vi "Pixel time analisis viewer.vi"() -> ()   [LabVIEW 2015, in "VIPM2.lvlib"]
uses:
  VIPM2.lvlib
  <vilib>/Analysis/NI_AALBase.lvlib
panel:
  out "Integrated Last event (s)":dbl format="%#.4f s"
  out "Chip Last event (s)":dbl format="%#.4f s"
  out "Chip First event (s)":dbl format="%#.4f s"
  out "Global Last event (s)":dbl format="%#.4f s"
  out "Pixel":u8
  out "Integrated events":i32
  out "Global last event (hex)":u64 format="%.0x"
  out "Global 1st event (hex)":u64 format="%.0x"
  in  "Integration pointer slide":u64(slide) scale=143772870070.0..145064784669.0 scale format="%x"
  out "Total time bar":cluster{u64, u64}(slide) scale=141174816241.0..145064861029.0 scale format="%x"
  in  "Pixel":u8 max=99
  in  "Chip ID":u16 format="%04x"
  out "Barra Load events":i32(slide) scale=-1.0..40000.0
  in  "X scale max.":dbl=150.0 min=0.0 max=1e+29 step=10.0
  in  "X scale min.":dbl=80.0 min=0.0 max=1e+29 step=10.0
  in  "Y scale":dbl=100.0 min=5.0 max=1e+29 step=10.0
  in  "Take image button":bool
  in  "Close button":bool
  out "Total number of events":i32 caption="Total number of events\nCentrals"
  out "data time":string
  in  "ACQ full DATA file path":path caption="File path"
  out "Chip ID":string
  out "Trigger histogram 08":T1(graph)
  out "Trigger histogram 07":T1(graph)
  out "Trigger histogram 06":T1(graph)
  out "Trigger histogram 01":T1(graph)
  out "Trigger histogram 02":T1(graph)
  out "Trigger histogram 03":T1(graph)
  out "Trigger histogram 04":T1(graph)
  out "Trigger histogram 00":T1(graph)
  out "Trigger histogram 05":T1(graph)
  # "Global acquisition time"
  # "03"
  # "04"
  # "05"
  # "Global First acquired event"
  # "Global Last acquired event"
  # "This Chip First event"
  # "This Chip Last event"
  # "02"
  # "00"
  # "01"
  # "Integration slide"
  # "Last integrated event"
  # "08"
  # "07"
  # "06"
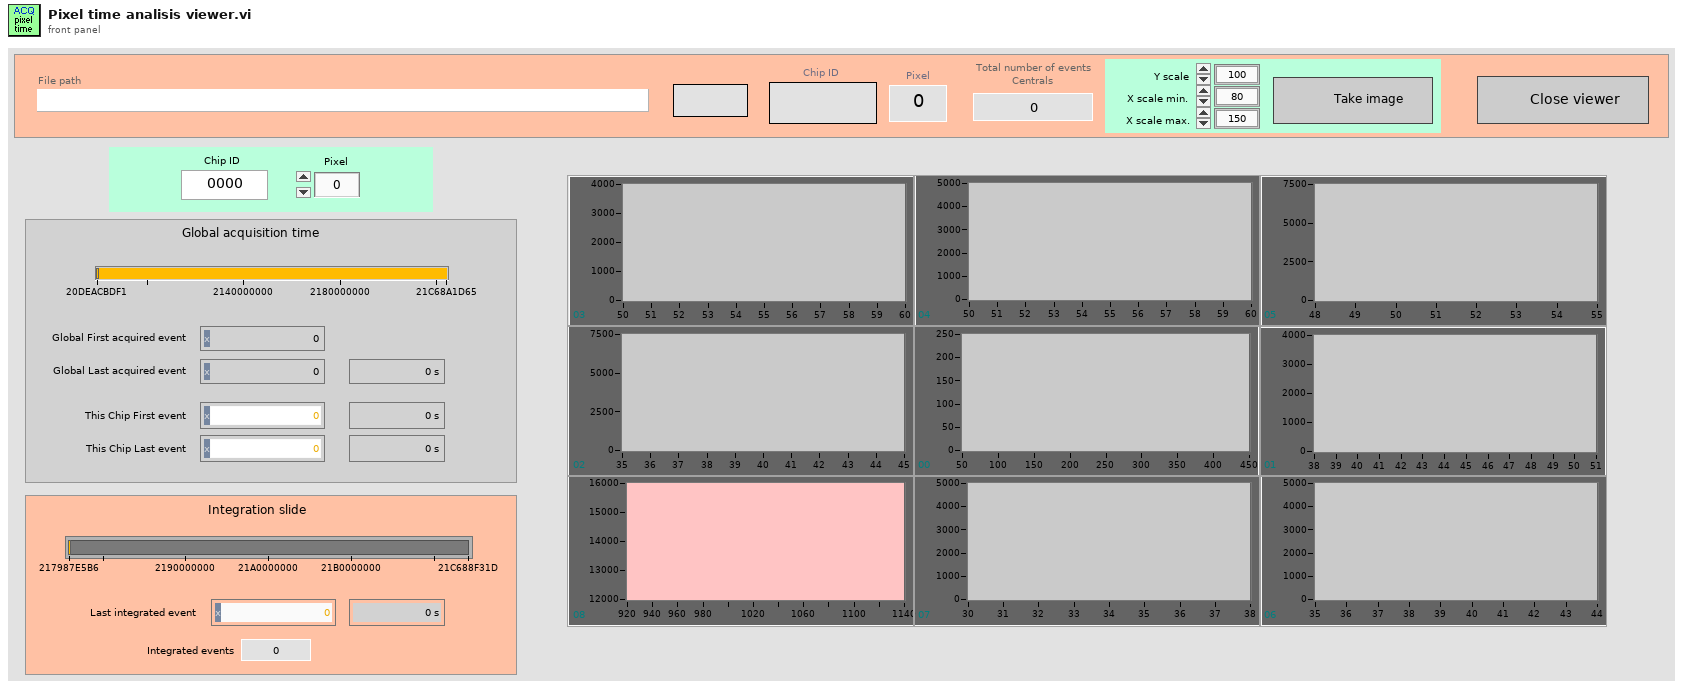
[diagram p1: front panel]
types:
  T1 = cluster{"X Values":dbl[], "Histogram: h(x)":i32[]}
  T2 = enum16{"big-endian, network order", "native, host order", "little-endian"}
  T3 = typedef "imagedata.ctl" = cluster{"image type":i32, "image depth":i32, "image":u8[], "mask":u8[], "colors":u32[], "Rectangle":cluster{"left":i16, "top":i16, "right":i16, "bottom":i16}}
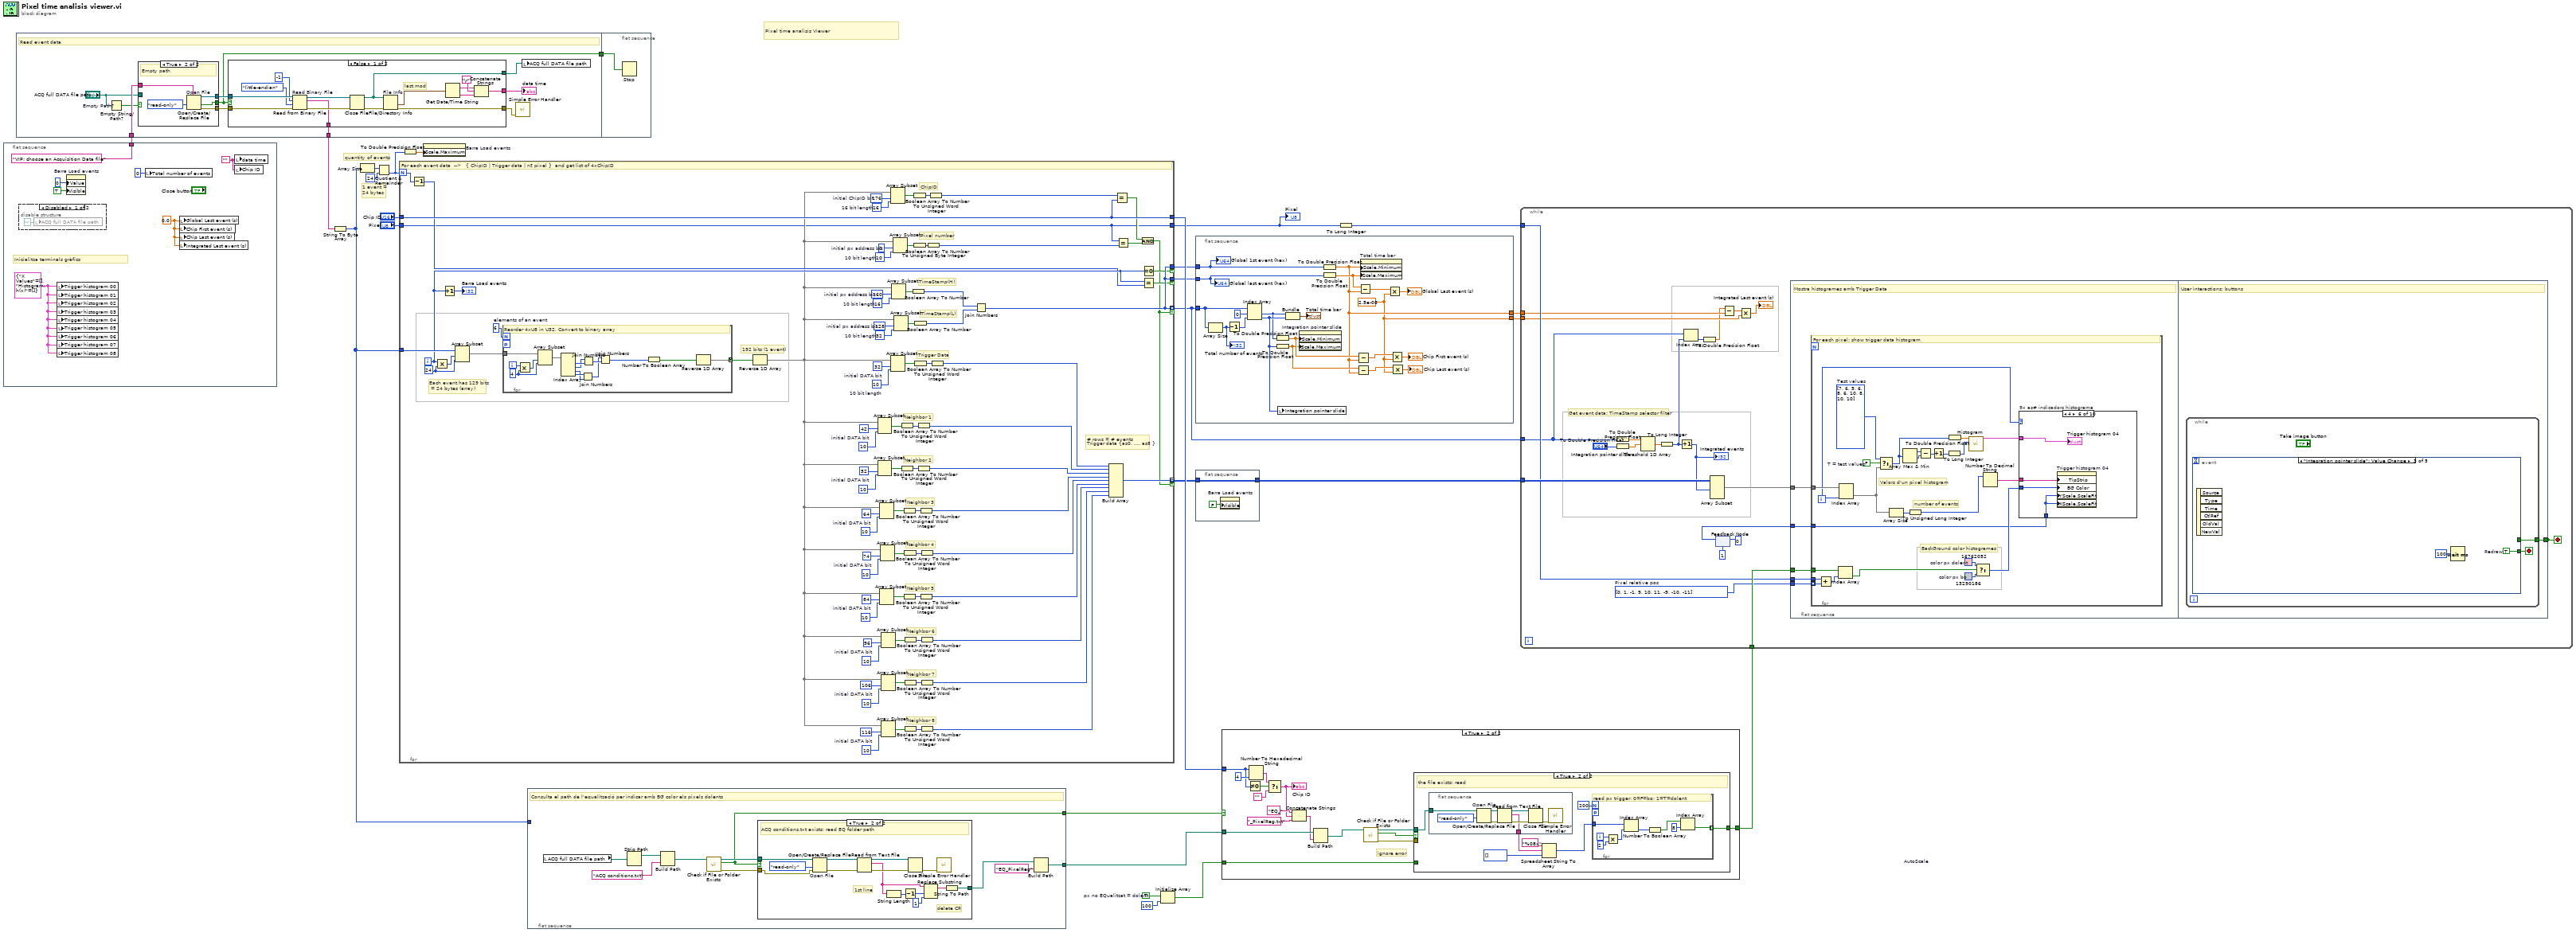
[diagram p0: block diagram]
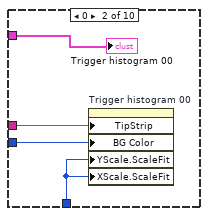
[diagram p3: hidden frame]
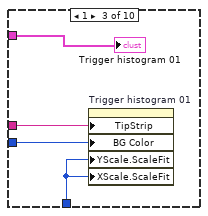
[diagram p4: hidden frame]
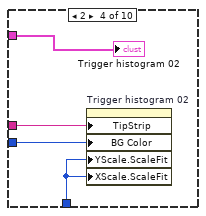
[diagram p5: hidden frame]
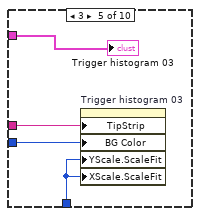
[diagram p6: hidden frame]
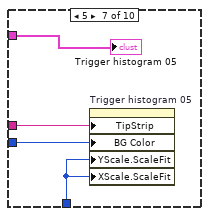
[diagram p7: hidden frame]
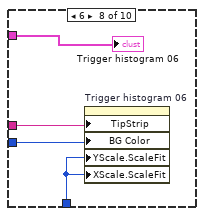
[diagram p8: hidden frame]
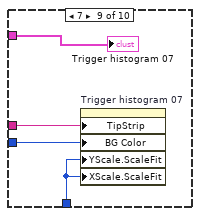
[diagram p9: hidden frame]
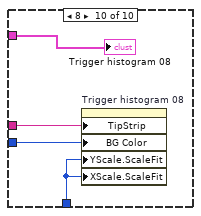
[diagram p10: hidden frame]
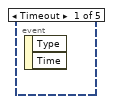
[diagram p11: hidden frame]
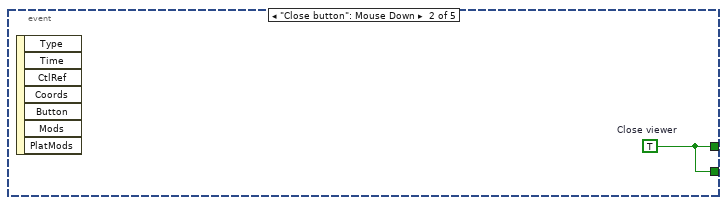
[diagram p12: hidden frame]
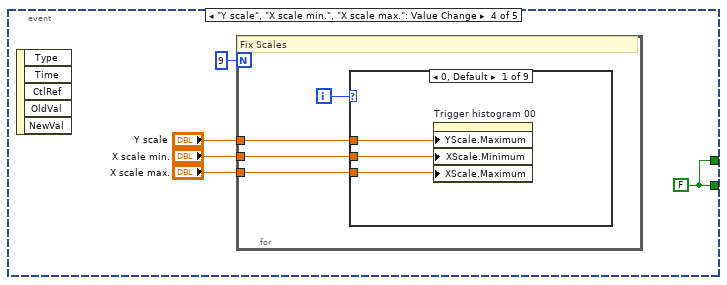
[diagram p13: hidden frame]
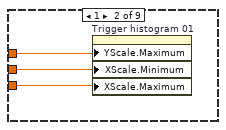
[diagram p14: hidden frame]
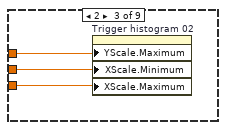
[diagram p15: hidden frame]
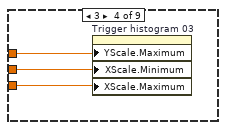
[diagram p16: hidden frame]
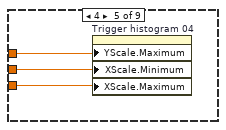
[diagram p17: hidden frame]
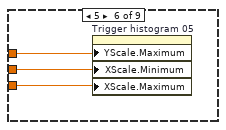
[diagram p18: hidden frame]
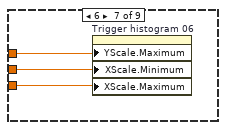
[diagram p19: hidden frame]
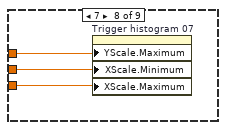
[diagram p20: hidden frame]
diagram:
  w16 = TRUE  # px no EQualitzat = dolent
  # "1 event =\n24 bytes"
  # "quantity of events"
  # "Pixel time analisis Viewer"
  n1 = flat-sequence {
    tunnel: ["VIP: choose an Acquisition Data file" ("prompt")] -> w25
    frame #0 {
      w27 = 0.0 ("Global Last event (s)")
      w28 = T1 {"X Values"=[], "Histogram: h(x)"=[]} ("Trigger histogram 00")
      w32 = ""
      # "Inicialitza terminals gràfics"
      n2 = disable-structure shown="Disabled" {
        frame Disabled {
          n3 = local write "ACQ full DATA file path"(path "") -> ()
        }
        frame Enabled {
        }
      }
      n4 = local write "Trigger histogram 00"(w28) -> ()
      n5 = local write "Trigger histogram 01"(w28) -> ()
      n6 = local write "Trigger histogram 02"(w28) -> ()
      n7 = local write "Trigger histogram 03"(w28) -> ()
      n8 = local write "Trigger histogram 04"(w28) -> ()
      n9 = local write "Trigger histogram 05"(w28) -> ()
      n10 = local write "Trigger histogram 06"(w28) -> ()
      n11 = local write "Trigger histogram 07"(w28) -> ()
      n12 = local write "Trigger histogram 08"(w28) -> ()
      n13 = property on="Barra Load events" class="Slide (strict)"("Value"=0 ("Barra Load events"), "Visible"=TRUE) -> ()  [unwired: 2 in, 2 out]
      n14 = local write "Total number of events"(0 ("Total number of events")) -> ()
      n15 = local write "Global Last event (s)"(w27) -> ()
      n16 = local write "Chip First event (s)"(w27) -> ()
      n17 = local write "Chip Last event (s)"(w27) -> ()
      n18 = local write "Integrated Last event (s)"(w27) -> ()
      n19 = local write "data time"(w32) -> ()
      n20 = local write "Chip ID"(w32) -> ()
    }
  }
  n21 = flat-sequence {
    tunnel: w25 -> [w41]
    tunnel: [w38] -> w22
    tunnel: [w36] -> w13
    tunnel: w13 -> [w72]
    frame #0 {
      # "Read event data"
      n22 = Empty String/Path? "Empty Path?"(string/path="ACQ full DATA file path") -> (empty?=w40:bool)
      n23 = case shown="True" w40 {
        tunnel: [w47 w52] -> w44
        tunnel: [w46 w51] -> w43
        tunnel: [_ w50] -> w36
        tunnel: w41 -> [_ w49]
        tunnel: "ACQ full DATA file path" -> [w45 _]
        frame False {
          # "Path input"
          n24 = Open/Create/Replace File "Open File"(file path (use dialog)=w45, access (0:read/write)=enum16{"read/write", "read-only", "write-only"}."read-only") -> (refnum out=w46:refnum<file>, error out=w47:errorcluster)  [unwired: 4 in, 1 out]
        }
        frame True {
          # "Empty path"
          n25 = Open/Create/Replace File "Open File"(prompt=w49, access (0:read/write)=enum16{"read/write", "read-only", "write-only"}."read-only") -> (refnum out=w51:refnum<file>, cancelled=w50:bool, error out=w52:errorcluster)  [unwired: 4 in]
        }
      }
      n26 = case shown="False" w36 {
        tunnel: w44 -> [w68 w71]
        tunnel: w43 -> [w67 w70]
        tunnel: [w62 _] -> w38
        tunnel: [w56 _] -> w42
        tunnel: [w55 _] -> w37
        tunnel: [w54 w69] -> w35
        frame False {
          # "last mod"
          n27 = Read from Binary File "Read Binary File"(8:w68, 9:T2."little-endian" ("byte order (0:big-endian, network order)"), 10:-1 ("count (1)"), 11:w67) -> (0:w65:errorcluster, 2:w62:string, 3:w64:refnum<file>)  [unwired: 2 in, 1 out]
          n28 = Close File(refnum=w64, error in=w65) -> (path=w55:path, error out=w61:errorcluster)
          n29 = File/Directory Info "File Info"(path=w55, error in=w61) -> (last mod=w57:timestamp, error out=w54:errorcluster)  [unwired: 5 out]
          n30 = Get Date/Time String(seconds (now)=w57) -> (date string=w58:string, time string=w60:string)  [unwired: 2 in]
          n31 = Concatenate Strings(w58, "\r", w60) -> (w56:string)
        }
        frame True {
          # "Cancelled openning"
          n32 = Close File(refnum=w70, error in=w71) -> (error out=w69:errorcluster)  [unwired: 1 out]
        }
      }
      "data time" <- w42
      n33 = call <vilib>:"Simple Error Handler.vi"("error in (no error)"=w35) -> ()  [unwired: 4 in, 5 out]
      n34 = local write "ACQ full DATA file path"(w37) -> ()
    }
    frame #1 {
      n35 = Stop(stop? (T)=w72) -> ()
    }
  }
  n36 = String To Byte Array(string=w22) -> (unsigned byte array=w1:u8[])
  n37 = Array Size(array=w1) -> (size(s)=w23:i32)
  n38 = Quotient & Remainder(x=w23, y=24) -> (floor(x/y)=w20:i32)  [unwired: 1 out]
  n39 = for {
    N: w20 -> [w77]
    tunnel: w1 -> [w151]
    tunnel: [w136] -> w18 mode=indexing if=w74
    tunnel: "Chip ID" -> [w102]
    tunnel: [w102] -> w26
    tunnel: "Pixel" -> [w73]
    tunnel: [w81] -> w10 mode=indexing if=w74
    tunnel: [w81] -> w11 if=w79
    tunnel: [w81] -> w12 if=w80
    tunnel: [w73] -> w4
    i -> [w78]
    w85 = 16  # 10 bit length
    w86 = 160  # initial px address bit
    w88 = 32  # 10 bit length
    w87 = 128  # initial px address bit
    w106 = 116  # initial DATA bit
    w110 = 106  # initial DATA bit
    w114 = 96  # initial DATA bit
    w118 = 84  # initial DATA bit
    w122 = 74  # initial DATA bit
    w126 = 64  # initial DATA bit
    w130 = 52  # initial DATA bit
    w134 = 42  # initial DATA bit
    w140 = 10  # 10 bit length
    w141 = 0  # initial px address bit
    w145 = 10  # 10 bit length
    w144 = 32  # initial DATA bit
    w148 = 16  # 16 bit length
    w149 = 176  # initial ChipID bit
    w154 = 24 ("y")
    w155 = 6  # elements of an event
    # "# rows = # events\nTrigger data {as0, ..., as8 }"
    # "TimeStamp(H)"
    # "TimeStamp(L)"
    # "Neighbor 8"
    # "Neighbor 7"
    # "Neighbor 6"
    # "Neighbor 5"
    # "Neighbor 4"
    # "Neighbor 3"
    # "Neighbor 2"
    # "Neighbor 1"
    # "Pixel number"
    # "Trigger Data"
    # "ChipID"
    # "192 bits (1 event)"
    # "Each event has 129 bits\n = 24 bytes (array)"
    # "For each event data  -->   { ChipID | Trigger data | nº pixel }  and get list of 4xChipID"
    n40 = Decrement(x=w77) -> (x-1=w76:i32)
    n41 = Multiply(x=w78, y=w154) -> (x*y=w153:i32)
    n42 = Increment(x=w78) -> (x+1=→"Barra Load events":i32)
    n43 = Array Subset "Array Subset"(array=w151, index=w153, length=w154) -> (w152:u8[])
    n44 = for {
      N: w155 -> [_]
      tunnel: w152 -> [w168]
      workers-P: _ -> [_]
      tunnel: [w156] -> w150 mode=concatenating
      i -> [w169]
      w166 = 4 ("y")
      # "Reorder 4xU8 in U32. Convert to binary array"
      n45 = Multiply(x=w169, y=w166) -> (x*y=w167:i32)
      n46 = Array Subset "Array Subset"(array=w168, index=w167, length=w166) -> (w165:u8[])
      n47 = Index Array(array=w165) -> (element #1=w164:u8, element #2=w163:u8, element #3=w161:u8, element #4=w162:u8)  [unwired: 4 in]
      n48 = Join Numbers(hi=w162, lo=w161) -> ((hi.lo)=w159:u16)
      n49 = Join Numbers(hi=w163, lo=w164) -> ((hi.lo)=w160:u16)
      n50 = Join Numbers(hi=w159, lo=w160) -> ((hi.lo)=w157:u32)
      n51 = Number To Boolean Array(number=w157) -> (Boolean array=w158:bool[])
      n52 = Reverse 1D Array(array=w158) -> (reversed array=w156:bool[])
    }
    n53 = Reverse 1D Array(array=w150) -> (reversed array=w75:bool[])
    n54 = Array Subset "Array Subset"(array=w75, index=w134, length=10 ("10 bit length")) -> (w132:bool[])
    n55 = Array Subset "Array Subset"(array=w75, index=w130, length=10 ("10 bit length")) -> (w128:bool[])
    n56 = Array Subset "Array Subset"(array=w75, index=w126, length=10 ("10 bit length")) -> (w124:bool[])
    n57 = Array Subset "Array Subset"(array=w75, index=w118, length=10 ("10 bit length")) -> (w116:bool[])
    n58 = Array Subset "Array Subset"(array=w75, index=w122, length=10 ("10 bit length")) -> (w120:bool[])
    n59 = Array Subset "Array Subset"(array=w75, index=w114, length=10 ("10 bit length")) -> (w112:bool[])
    n60 = Array Subset "Array Subset"(array=w75, index=w110, length=10 ("10 bit length")) -> (w108:bool[])
    n61 = Array Subset "Array Subset"(array=w75, index=w106, length=10 ("10 bit length")) -> (w104:bool[])
    n62 = Array Subset "Array Subset"(array=w75, index=w149, length=w148) -> (w147:bool[])
    n63 = Array Subset "Array Subset"(array=w75, index=w144, length=w145) -> (w142:bool[])
    n64 = Array Subset "Array Subset"(array=w75, index=w86, length=w85) -> (w84:bool[])
    n65 = Array Subset "Array Subset"(array=w75, index=w141, length=w140) -> (w139:bool[])
    n66 = Array Subset "Array Subset"(array=w75, index=w87, length=w88) -> (w89:bool[])
    n67 = Boolean Array To Number(Boolean array=w132) -> (number=w133:u32)
    n68 = Boolean Array To Number(Boolean array=w128) -> (number=w129:u32)
    n69 = Boolean Array To Number(Boolean array=w124) -> (number=w125:u32)
    n70 = Boolean Array To Number(Boolean array=w116) -> (number=w117:u32)
    n71 = Boolean Array To Number(Boolean array=w120) -> (number=w121:u32)
    n72 = Boolean Array To Number(Boolean array=w112) -> (number=w113:u32)
    n73 = Boolean Array To Number(Boolean array=w108) -> (number=w109:u32)
    n74 = Boolean Array To Number(Boolean array=w104) -> (number=w105:u32)
    n75 = Boolean Array To Number(Boolean array=w84) -> (number=w82:u32)
    n76 = Boolean Array To Number(Boolean array=w147) -> (number=w146:u32)
    n77 = Boolean Array To Number(Boolean array=w139) -> (number=w138:u32)
    n78 = Boolean Array To Number(Boolean array=w89) -> (number=w83:u32)
    n79 = Boolean Array To Number(Boolean array=w142) -> (number=w143:u32)
    n80 = To Unsigned Word Integer(number=w133) -> (unsigned 16bit integer=w97:u16)
    n81 = To Unsigned Word Integer(number=w129) -> (unsigned 16bit integer=w96:u16)
    n82 = To Unsigned Word Integer(number=w125) -> (unsigned 16bit integer=w95:u16)
    n83 = To Unsigned Word Integer(number=w117) -> (unsigned 16bit integer=w93:u16)
    n84 = To Unsigned Word Integer(number=w121) -> (unsigned 16bit integer=w94:u16)
    n85 = To Unsigned Word Integer(number=w113) -> (unsigned 16bit integer=w92:u16)
    n86 = To Unsigned Word Integer(number=w109) -> (unsigned 16bit integer=w91:u16)
    n87 = To Unsigned Word Integer(number=w105) -> (unsigned 16bit integer=w90:u16)
    n88 = To Unsigned Byte Integer(number=w138) -> (unsigned 8bit integer=w101:u8)
    n89 = To Unsigned Word Integer(number=w146) -> (unsigned 16bit integer=w103:u16)
    n90 = To Unsigned Word Integer(number=w143) -> (unsigned 16bit integer=w98:u16)
    n91 = Join Numbers(hi=w82, lo=w83) -> ((hi.lo)=w81:u64)
    n92 = Build Array "Build Array"(w98, w97, w96, w95, w94, w93, w92, w91, w90) -> (w136:u16[])
    n93 = Equal?(x=w103, y=w102) -> (x = y?=w99:bool)
    n94 = Equal?(x=w73, y=w101) -> (x = y?=w100:bool)
    n95 = And(x=w99, y=w100) -> (x .and. y?=w74:bool)
    n96 = Equal To 0?(x=w78) -> (x = 0?=w80:bool)
    n97 = Equal?(x=w78, y=w76) -> (x = y?=w79:bool)
  }
  "Pixel" <- w4
  n98 = To Double Precision Float(number=w20) -> (double precision float=w21:dbl)
  n99 = property on="Barra Load events" class="Slide (strict)"("Scale.Maximum"=w21) -> ()  [unwired: 2 in, 2 out]
  n100 = flat-sequence {
    tunnel: [w170] -> w8
    tunnel: [w173] -> w9
    tunnel: w1 -> [_]
    frame #0 {
      # "Consulta el path de l'equalització per indicar amb BG color els pixels dolents"
      n101 = local read "ACQ full DATA file path"() -> (w174:path)
      n102 = Strip Path(path=w174) -> (stripped path=w175:path)  [unwired: 1 out]
      n103 = Build Path(base path=w175, name or relative path="ACQ conditions.txt") -> (appended path=w177:path)
      n104 = call <vilib>:"Check if File or Folder Exists.vi"("path"=w177) -> ("error out"=w179:errorcluster, "file or folder exists?"=w173:bool, "dup path"=w178:path)  [unwired: 8 in]
      n105 = case shown="True" w173 {
        tunnel: w178 -> [_ w193]
        tunnel: w179 -> [_ w191]
        tunnel: [_ w180] -> w171
        frame False {
          # "ACQ conditions.txt doesn't exist"
        }
        frame True {
          # "delete CR"
          # "1st line"
          # "ACQ conditions.txt exists: read EQ folder path"
          n106 = Open/Create/Replace File "Open File"(file path (use dialog)=w193, error in=w191, access (0:read/write)=enum16{"read/write", "read-only", "write-only"}."read-only") -> (refnum out=w190:refnum<file>, error out=w189:errorcluster)  [unwired: 3 in, 1 out]
          n107 = Read from Text File(file (use dialog)=w190, error in=w189) -> (refnum out=w188:refnum<file>, text=w181:string, error out=w187:errorcluster)  [unwired: 2 in, 1 out]
          n108 = String Length(string=w181) -> (length=w185:i32)
          n109 = Decrement(x=w185) -> (x-1=w184:i32)
          n110 = Close File(refnum=w188, error in=w187) -> (error out=w186:errorcluster)  [unwired: 1 out]
          n111 = Replace Substring(2:1 ("length (len. of substring)"), 3:w184, 5:w181) -> (1:w182:string)  [unwired: 1 in, 1 out]
          n112 = call <vilib>:"Simple Error Handler.vi"("error in (no error)"=w186) -> ()  [unwired: 4 in, 5 out]
          n113 = String To Path(string=w182) -> (path=w180:path)
        }
      }
      n114 = Build Path(base path=w171, name or relative path="EQ_PixelReg") -> (appended path=w170:path)
    }
  }
  n115 = Initialize Array "Initialize Array"(w16, 100 ("dimension size")) -> (w7:bool[])
  n116 = flat-sequence {
    tunnel: w12 -> [w209]
    tunnel: w11 -> [w208]
    tunnel: w10 -> [w212]
    tunnel: [w195] -> w3
    tunnel: [w194] -> w2
    frame #0 {
      w194 = 2.5e-08 ("y")
      n117 = Array Size(array=w212) -> (size(s)=w207:i32)
      "Total number of events" <- w207
      n118 = Decrement(x=w207) -> (x-1=w211:i32)
      n119 = Index Array "Index Array"(array=w212, index #1=0 ("index"), index #2=w211) -> (element #1=w205:u64, element #2=w206:u64)
      n120 = To Double Precision Float(number=w205) -> (double precision float=w199:dbl)
      n121 = To Double Precision Float(number=w206) -> (double precision float=w197:dbl)
      n122 = local write "Integration pointer slide"(w206) -> ()
      n123 = Bundle(w205, w206) -> (→"Total time bar":cluster{u64, u64})  [unwired: 1 in]
      n124 = property on="Integration pointer slide" class="Slide (strict)"("Scale.Minimum"=w199, "Scale.Maximum"=w197) -> ()  [unwired: 2 in, 2 out]
      n125 = To Double Precision Float(number=w209) -> (double precision float=w195:dbl)
      n126 = To Double Precision Float(number=w208) -> (double precision float=w204:dbl)
      n127 = Subtract(x=w199, y=w195) -> (x-y=w198:dbl)
      n128 = Subtract(x=w197, y=w195) -> (x-y=w196:dbl)
      n129 = Subtract(x=w204, y=w195) -> (x-y=w203:dbl)
      n130 = property on="Total time bar" class="Slide (strict)"("Scale.Minimum"=w195, "Scale.Maximum"=w204) -> ()  [unwired: 2 in, 2 out]
      n131 = Multiply(x=w203, y=w194) -> (x*y=→"Global Last event (s)":dbl)
      n132 = Multiply(x=w198, y=w194) -> (x*y=→"Chip First event (s)":dbl)
      n133 = Multiply(x=w196, y=w194) -> (x*y=→"Chip Last event (s)":dbl)
      "Global 1st event (hex)" <- w209
      "Global last event (hex)" <- w208
    }
  }
  n134 = flat-sequence {
    tunnel: [w215] -> w19
    tunnel: w18 -> [w215]
    frame #0 {
      n135 = property on="Barra Load events" class="Slide (strict)"("Visible"=FALSE) -> ()  [unwired: 2 in, 2 out]
    }
  }
  n136 = case shown="True" w9 {
    tunnel: w8 -> [_ w232]
    tunnel: [w216 w224] -> w6
    tunnel: w7 -> [w216 w223]
    tunnel: w26 -> [_ w217]
    frame False {
    }
    frame True {
      # "ignore error"
      n137 = Not Equal To 0?(x=w217) -> (x != 0?=w221:bool)
      n138 = Number To Hexadecimal String(1:i16 4 ("width (-)"), 2:w217) -> (0:w220:string)
      n139 = Select(t=w220, s=w221, f="") -> (s? t:f=w218:string)
      "Chip ID" <- w218
      n140 = Concatenate Strings "Concatenate Strings"("EQ_", w218, "_PixelReg.txt") -> (w229:string)
      n141 = Build Path(base path=w232, name or relative path=w229) -> (appended path=w228:path)
      n142 = call <vilib>:"Check if File or Folder Exists.vi"("path"=w228) -> ("error out"=w225:errorcluster, "file or folder exists?"=w226:bool, "dup path"=w227:path)  [unwired: 8 in]
      n143 = case shown="True" w226 {
        tunnel: w227 -> [_ w240]
        tunnel: w225 -> [_ _]
        tunnel: [w233 w234] -> w224
        tunnel: w223 -> [w233 _]
        frame False {
          # "the file does not exist: do not do anything"
        }
        frame True {
          # "the file exists: read"
          n144 = flat-sequence {
            tunnel: w240 -> [w256]
            tunnel: [w249] -> w239
            frame #0 {
              n145 = Open/Create/Replace File "Open File"(file path (use dialog)=w256, access (0:read/write)=enum16{"read/write", "read-only", "write-only"}."read-only") -> (refnum out=w253:refnum<file>, error out=w254:errorcluster)  [unwired: 4 in, 1 out]
              n146 = Read from Text File(file (use dialog)=w253, error in=w254) -> (refnum out=w252:refnum<file>, text=w249:string, error out=w251:errorcluster)  [unwired: 2 in, 1 out]
              n147 = Close File(refnum=w252, error in=w251) -> (error out=w250:errorcluster)  [unwired: 1 out]
              n148 = call <vilib>:"Simple Error Handler.vi"("error in (no error)"=w250) -> ()  [unwired: 4 in, 5 out]
            }
          }
          n149 = Spreadsheet String To Array(format string="%08x", spreadsheet string=w239, array type (2D Dbl)=u32[] []) -> (array=w236:u32[])  [unwired: 1 in]
          n150 = for {
            N: 200 -> [_]
            tunnel: w236 -> [w245]
            tunnel: [w241] -> w234 mode=indexing
            workers-P: _ -> [_]
            i -> [w248]
            # "read px trigger: 0=F=bo; 1=T=dolent"
            n151 = Multiply(x=w248, y=2) -> (x*y=w246:i32)
            n152 = Index Array "Index Array"(array=w245, index=w246) -> (element=w244:u32)
            n153 = Number To Boolean Array(number=w244) -> (Boolean array=w243:bool[])
            n154 = Index Array "Index Array"(array=w243, index=8) -> (element=w241:bool)
          }
        }
      }
    }
  }
  n155 = To Long Integer(number=w4) -> (32bit integer=w5:i32)
  n156 = while {
    tunnel: w19 -> [w274]
    tunnel: w10 -> [w265]
    tunnel: w5 -> [w270]
    tunnel: w6 -> [w272]
    tunnel: w3 -> [w262]
    tunnel: w2 -> [w260]
    stop <- w269 stop-if-true
    w271 = i32[] [0, 1, -1, 9, 10, 11, -9, -10, -11]  # Pixel relative pos
    # "Get event data: TimeStamp selector filter"
    n157 = To Double Precision Float(number=w265) -> (double precision float=w276:dbl[])
    n158 = To Double Precision Float(number="Integration pointer slide") -> (double precision float=w278:dbl)
    n159 = Threshold 1D Array(2:w278, 3:w276) -> (0:w275:dbl)  [unwired: 1 in]
    n160 = To Long Integer(number=w275) -> (32bit integer=w257:i32)
    n161 = Increment(x=w257) -> (x+1=w264:i32)
    "Integrated events" <- w264
    n162 = Index Array "Index Array"(array=w265, index=w257) -> (element=w263:u64)
    n163 = To Double Precision Float(number=w263) -> (double precision float=w259:dbl)
    n164 = Array Subset "Array Subset"(array=w274, length (row)=w264) -> (w273:u16[][])  [unwired: 3 in]
    n165 = feedback #1 "AutoScale"(u8 1 ("X Scale.Scale Fit")) -> (w266:u8)
    n166 = feedback-in #1(u8 0 ("X Scale.Scale Fit")) -> ()
    n167 = Subtract(x=w259, y=w262) -> (x-y=w261:dbl)
    n168 = Multiply(x=w261, y=w260) -> (x*y=→"Integrated Last event (s)":dbl)
    n169 = flat-sequence {
      tunnel: w273 -> [w283]
      tunnel: w272 -> [w282]
      tunnel: w271 -> [w281]
      tunnel: w270 -> [w280]
      tunnel: w266 -> [w279]
      tunnel: [w345] -> _
      tunnel: [w345] -> w269
      frame #0 {
        # "Mostra histogrames amb Trigger Data"
        n170 = for {
          tunnel: w283 -> [w288]
          tunnel: w282 -> [w293]
          tunnel: w280 -> [w291]
          tunnel: w281 -> [w290] mode=indexing
          tunnel: w279 -> [w284]
          i -> [w286]
          w295 = u32 13290186  # color px bo
          w294 = u32 16762052  # color px dolent
          w300 = u16[] [7, 6, 5, 6, 8, 6, 10, 8, 10, 10]  # Test values
          w299 = FALSE  # T = test values
          # "BackGround color histogrames"
          # "number of events"
          # "Valors d'un pixel histogram"
          # "For each pixel: show trigger data histogram"
          n171 = Add(x=w291, y=w290) -> (x+y=w292:i32)
          n172 = Index Array "Index Array"(array=w293, index=w292) -> (element=w289:bool)
          n173 = Index Array "Index Array"(array=w288, index (col)=w286) -> (element=w287:u16[])  [unwired: 1 in]
          n174 = Select(t=w300, s=w299, f=w287) -> (s? t:f=w301:u16[])
          n175 = Array Size(array=w287) -> (size(s)=w298:i32)
          n176 = Array Max & Min(array=w301) -> (max value=w305:u16, min value=w304:u16)  [unwired: 2 out]
          n177 = To Unsigned Long Integer(number=w298) -> (unsigned 32bit integer=w297:u32)
          n178 = Subtract(x=w305, y=w304) -> (x-y=w303:u16)
          n179 = Increment(x=w303) -> (x+1=w307:u16)
          n180 = To Long Integer(number=w307) -> (32bit integer=w308:i32)
          n181 = To Double Precision Float(number=w301) -> (double precision float=w306:dbl[])
          n182 = call <vilib>:"Histogram.vi"("intervals"=w308, "X"=w306) -> ("Histogram Graph"=w302:T1)  [unwired: 6 in, 3 out]
          n183 = Select(t=w294, s=w289, f=w295) -> (s? t:f=w285:u32)
          n184 = Number To Decimal String(number=w297) -> (decimal integer string=w296:string)  [unwired: 1 in]
          n185 = case "9x as# indicadors histograma" shown="4" w286 {
            tunnel: w302 -> [_ w312 w316 w320 w324 w328 w332 w336 w340 w344]
            tunnel: w296 -> [_ w311 w315 w319 w323 w327 w331 w335 w339 w343]
            tunnel: w285 -> [_ w310 w314 w318 w322 w326 w330 w334 w338 w342]
            tunnel: w284 -> [_ w309 w313 w317 w321 w325 w329 w333 w337 w341]
            frame Default {
            }
            frame 0 {
              n186 = property on="Trigger histogram 00" class="XYGraph (strict)"("TipStrip"=w311, "BG Color"=w310, "YScale.ScaleFit"=w309, "XScale.ScaleFit"=w309) -> ()  [unwired: 2 in, 2 out]
              "Trigger histogram 00" <- w312
            }
            frame 1 {
              n187 = property on="Trigger histogram 01" class="XYGraph (strict)"("TipStrip"=w315, "BG Color"=w314, "YScale.ScaleFit"=w313, "XScale.ScaleFit"=w313) -> ()  [unwired: 2 in, 2 out]
              "Trigger histogram 01" <- w316
            }
            frame 2 {
              n188 = property on="Trigger histogram 02" class="XYGraph (strict)"("TipStrip"=w319, "BG Color"=w318, "YScale.ScaleFit"=w317, "XScale.ScaleFit"=w317) -> ()  [unwired: 2 in, 2 out]
              "Trigger histogram 02" <- w320
            }
            frame 3 {
              n189 = property on="Trigger histogram 03" class="XYGraph (strict)"("TipStrip"=w323, "BG Color"=w322, "YScale.ScaleFit"=w321, "XScale.ScaleFit"=w321) -> ()  [unwired: 2 in, 2 out]
              "Trigger histogram 03" <- w324
            }
            frame 4 {
              n190 = property on="Trigger histogram 04" class="XYGraph (strict)"("TipStrip"=w327, "BG Color"=w326, "YScale.ScaleFit"=w325, "XScale.ScaleFit"=w325) -> ()  [unwired: 2 in, 2 out]
              "Trigger histogram 04" <- w328
            }
            frame 5 {
              n191 = property on="Trigger histogram 05" class="XYGraph (strict)"("TipStrip"=w331, "BG Color"=w330, "YScale.ScaleFit"=w329, "XScale.ScaleFit"=w329) -> ()  [unwired: 2 in, 2 out]
              "Trigger histogram 05" <- w332
            }
            frame 6 {
              n192 = property on="Trigger histogram 06" class="XYGraph (strict)"("TipStrip"=w335, "BG Color"=w334, "YScale.ScaleFit"=w333, "XScale.ScaleFit"=w333) -> ()  [unwired: 2 in, 2 out]
              "Trigger histogram 06" <- w336
            }
            frame 7 {
              n193 = property on="Trigger histogram 07" class="XYGraph (strict)"("TipStrip"=w339, "BG Color"=w338, "YScale.ScaleFit"=w337, "XScale.ScaleFit"=w337) -> ()  [unwired: 2 in, 2 out]
              "Trigger histogram 07" <- w340
            }
            frame 8 {
              n194 = property on="Trigger histogram 08" class="XYGraph (strict)"("TipStrip"=w343, "BG Color"=w342, "YScale.ScaleFit"=w341, "XScale.ScaleFit"=w341) -> ()  [unwired: 2 in, 2 out]
              "Trigger histogram 08" <- w344
            }
          }
        }
      }
      frame #1 {
        # "User interactions: buttons"
        n195 = while {
          tunnel: [w347] -> w345
          stop <- w346 stop-if-true
          n196 = event shown="[2] \"Integration pointer slide\": Value Change" {
            selector: _ -> [_ _ _ _ _]
            dyn-events: _ -> [_ _ _ _ _]
            timeout: _ -> [_ _ _ _ _]
            tunnel: [_ w348 _ w355 w387] -> w347
            tunnel: [_ w348 w350 w355 w387] -> w346
            event Timeout {
              n197 = event-data() -> ()  [unwired: 1 in, 2 out]
            }
            event "Close button": Mouse Down {
              w348 = TRUE  # Close viewer
              n198 = event-data() -> ()  [unwired: 1 in, 7 out]
            }
            event "Integration pointer slide": Value Change {
              w350 = TRUE  # Redraw
              n199 = event-data() -> ()  [unwired: 1 in, 6 out]
              n200 = Wait (ms)(milliseconds to wait=u32 100) -> ()  [unwired: 1 out]
            }
            event "Y scale", "X scale min.", "X scale max.": Value Change {
              w355 = FALSE ("Close viewer")
              n201 = event-data() -> ()  [unwired: 1 in, 5 out]
              n202 = for {
                N: 9 -> [_]
                tunnel: "Y scale" -> [w358]
                tunnel: "X scale min." -> [w357]
                tunnel: "X scale max." -> [w356]
                i -> [w359]
                # "Fix Scales"
                n203 = case shown="0, Default" w359 {
                  tunnel: w358 -> [w362 w365 w368 w371 w374 w377 w380 w383 w386]
                  tunnel: w357 -> [w361 w364 w367 w370 w373 w376 w379 w382 w385]
                  tunnel: w356 -> [w360 w363 w366 w369 w372 w375 w378 w381 w384]
                  frame 0, Default {
                    n204 = property on="Trigger histogram 00" class="XYGraph (strict)"("YScale.Maximum"=w362, "XScale.Minimum"=w361, "XScale.Maximum"=w360) -> ()  [unwired: 2 in, 2 out]
                  }
                  frame 1 {
                    n205 = property on="Trigger histogram 01" class="XYGraph (strict)"("YScale.Maximum"=w365, "XScale.Minimum"=w364, "XScale.Maximum"=w363) -> ()  [unwired: 2 in, 2 out]
                  }
                  frame 2 {
                    n206 = property on="Trigger histogram 02" class="XYGraph (strict)"("YScale.Maximum"=w368, "XScale.Minimum"=w367, "XScale.Maximum"=w366) -> ()  [unwired: 2 in, 2 out]
                  }
                  frame 3 {
                    n207 = property on="Trigger histogram 03" class="XYGraph (strict)"("YScale.Maximum"=w371, "XScale.Minimum"=w370, "XScale.Maximum"=w369) -> ()  [unwired: 2 in, 2 out]
                  }
                  frame 4 {
                    n208 = property on="Trigger histogram 04" class="XYGraph (strict)"("YScale.Maximum"=w374, "XScale.Minimum"=w373, "XScale.Maximum"=w372) -> ()  [unwired: 2 in, 2 out]
                  }
                  frame 5 {
                    n209 = property on="Trigger histogram 05" class="XYGraph (strict)"("YScale.Maximum"=w377, "XScale.Minimum"=w376, "XScale.Maximum"=w375) -> ()  [unwired: 2 in, 2 out]
                  }
                  frame 6 {
                    n210 = property on="Trigger histogram 06" class="XYGraph (strict)"("YScale.Maximum"=w380, "XScale.Minimum"=w379, "XScale.Maximum"=w378) -> ()  [unwired: 2 in, 2 out]
                  }
                  frame 7 {
                    n211 = property on="Trigger histogram 07" class="XYGraph (strict)"("YScale.Maximum"=w383, "XScale.Minimum"=w382, "XScale.Maximum"=w381) -> ()  [unwired: 2 in, 2 out]
                  }
                  frame 8 {
                    n212 = property on="Trigger histogram 08" class="XYGraph (strict)"("YScale.Maximum"=w386, "XScale.Minimum"=w385, "XScale.Maximum"=w384) -> ()  [unwired: 2 in, 2 out]
                  }
                }
              }
            }
            event "Take image button": Mouse Down {
              w387 = FALSE
              n213 = event-data() -> ()  [unwired: 1 in, 7 out]
              n214 = flat-sequence {
                tunnel: [w389] -> w388
                tunnel: w388 -> [w399]
                frame #0 {
                  n215 = local read "ACQ full DATA file path"() -> (w395:path)
                  n216 = local read "Chip ID"() -> (w394:string)
                  n217 = Strip Path(path=w395) -> (stripped path=w392:path)  [unwired: 1 out]
                  n218 = Concatenate Strings(w394, "_ACQ_time.png" ("name or relative path")) -> (w390:string)
                  n219 = invoke class="VI" method="FP.Get Image"("image depth"=24 ("Image Depth")) -> ("image data"=w397:T3)  [unwired: 5 in, 5 out]
                  n220 = Build Path(base path=w392, name or relative path=w390) -> (appended path=w396:path)
                  n221 = call <vilib>:"Write PNG File.vi"("image data"=w397, "path to PNG file"=w396) -> ()  [unwired: 8 in, 2 out]
                  n222 = Concatenate Strings("Image saved\n", w390) -> (w389:string)
                }
                frame #1 {
                  n223 = call "MessageTimeOk.vi"("time (ms)"=2500, "missage"=w399) -> ()  [unwired: 4 in]
                }
              }
            }
          }
        }
      }
    }
  }
